vi "自定义菜单.vi"() -> ()   [LabVIEW 2018]
panel:
  out "项标识符":string
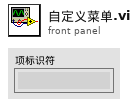
[diagram p1: front panel]
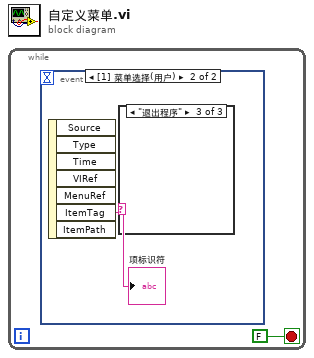
[diagram p0: block diagram]
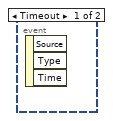
[diagram p2: hidden frame]
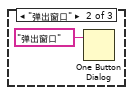
[diagram p4: hidden frame]
diagram:
  n1 = while {
    stop <- FALSE stop-if-true
    n2 = event shown="[1] 菜单选择(用户)" {
      selector: _ -> [_ _]
      dyn-events: _ -> [_ _]
      timeout: _ -> [_ _]
      event Timeout {
        n3 = event-data() -> ()  [unwired: 1 in, 3 out]
      }
      event Menu Selection (User) {
        n4 = event-data() -> ("ItemTag"=w2:string)  [unwired: 1 in, 6 out]
        "项标识符" <- w2
        n5 = case shown="\"退出程序\"" w2 {
          frame "假", Default {
          }
          frame "弹出窗口" {
            n6 = One Button Dialog(message="弹出窗口" ("消息")) -> ()  [unwired: 1 in, 1 out]
          }
          frame "退出程序" {
          }
        }
      }
    }
  }
